vi "Msg.vi"(7 "Actor in":refnum<class "Actor.lvclass">, 11 "Msg in":refnum<class "Msg.lvclass">) -> (0 "error out":errorcluster, 2 "Destroy Self?":bool, 5 "Actor out":refnum<class "Actor.lvclass">)   [LabVIEW 2021, in "AAM.lvlib" / "Msg.lvclass"]
uses:
  Msg.lvclass
  Actor/Actor.lvclass
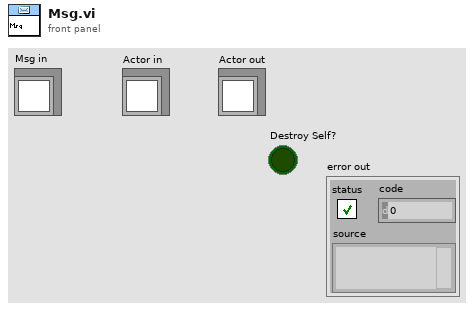
[diagram p1: front panel]
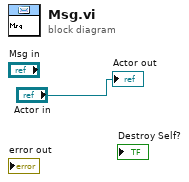
[diagram p0: block diagram]
diagram:
  "Actor out" <- "Actor in"
